vi "Slide Callback.vi"(7 "Owner":refnum<class>, 11 "Message":refnum<class "Message.lvclass">) -> (0 "error out":errorcluster)   [LabVIEW 2020]
uses:
  <vilib>/IlluminatedG/lv-msg-simple/Stream-Simple-Msg/Message/Message.lvclass
  56a5a06d-eb56-4e44-b9be-13e5cc0f8f90.vi
  <vilib>/IlluminatedG/lv-msg-simple/Stream-Simple-Msg/Message/Get Data.vi
  <vilib>/IlluminatedG/lv-msg-simple/Stream-Simple-Msg/Message/Flatten Type.vi
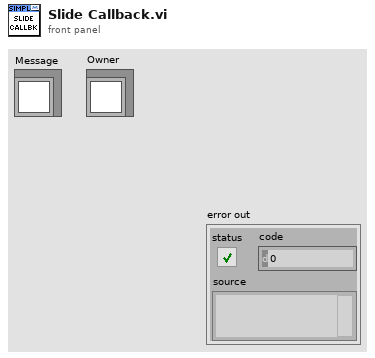
[diagram p1: front panel]
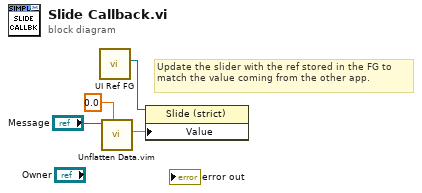
[diagram p0: block diagram]
diagram:
  # "Update the slider with the ref stored in the FG to match the value coming from the other app."
  n1 = call "UI Ref FG.vi"() -> ("Slide"=w3:refnum<vi>)  [unwired: 9 in, 2 out]
  n2 = call "Unflatten Data.vim"("Data Type (String)"=0.0, "Message in"="Message") -> ("Unflattened Data"=w2:dbl)  [unwired: 7 in, 2 out]
  n3 = property class="Slide (strict)"(reference=w3, "Value"=w2) -> ()  [unwired: 1 in, 2 out]
